vi "Setup voltage in.vi"(8 "error in (no error)":errorcluster, 10 "Run info in":T1, 11 "Sampling info in":T2={"Channels"=[], "Sampling freq"=0, "Output freq"=0, "Update freq"=0, "Steps per rev"=0, "Counts per rev"=0, "Amplifier"="", "Motor driver"="", "Step bit"=0, "Max speed"=0.0, "Max accel"=0.0, "Pos gain"=0.0, "Vel gain"=0.0, "counter"="Dev1/ctr0"} {"Channels"."Hi cutoff" items=["500"=500.0, "1k"=1000.0, "5k"=5000.0, "10k"=10000.0, "20k"=20000.0]; "Channels"."Lo cutoff" items=["0.1"=0.1, "1"=1.0, "10"=10.0, "100"=100.0, "300"=300.0]; "Channels"."Gain" items=["x100"=100, "x1000"=1000, "x10000"=10000]}) -> (0 "error out":errorcluster, 2 "Run info":T1, 3 "Sampling info out":T2={"Channels"=[], "Sampling freq"=0, "Output freq"=0, "Update freq"=0, "Steps per rev"=0, "Counts per rev"=0, "Amplifier"="", "Motor driver"="", "Step bit"=0, "Max speed"=0.0, "Max accel"=0.0, "Pos gain"=0.0, "Vel gain"=0.0, "counter"="Dev1/ctr0"} {"Channels"."Hi cutoff" items=["500"=500.0, "1k"=1000.0, "5k"=5000.0, "10k"=10000.0, "20k"=20000.0]; "Channels"."Lo cutoff" items=["0.1"=0.1, "1"=1.0, "10"=10.0, "100"=100.0, "300"=300.0]; "Channels"."Gain" items=["x100"=100, "x1000"=1000, "x10000"=10000]})   [LabVIEW 2012]
uses:
  Sampling info.ctl
  Channel.ctl
  Run info.ctl
  <vilib>/DAQmx/configure/timing.llb/DAQmx Timing (Sample Clock).vi
  <vilib>/DAQmx/create/channels.llb/DAQmx Create Channel (AI-Voltage-Basic).vi
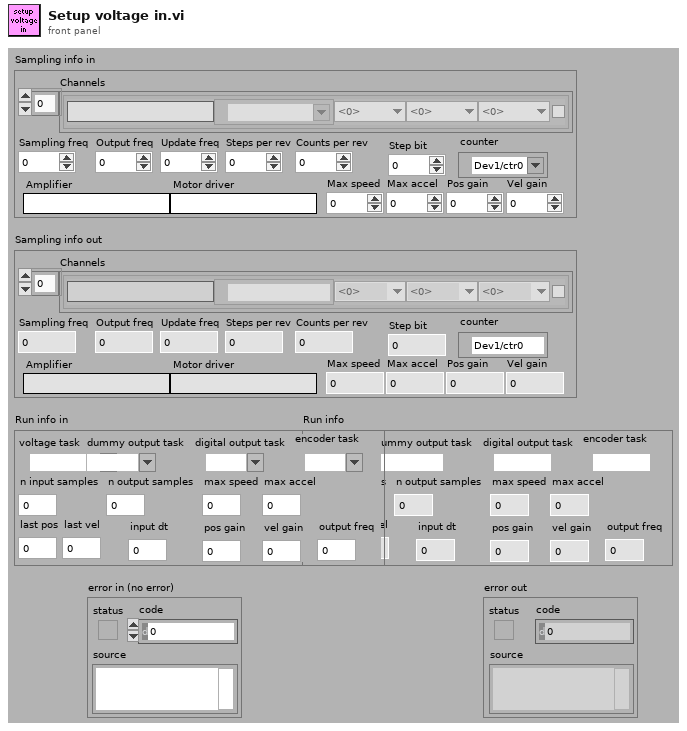
[diagram p1: front panel]
types:
  T1 = typedef "Run info.ctl" = cluster{"voltage task":refnum<k21>, "dummy output task":refnum<k21>, "digital output task":refnum<k21>, "encoder task":refnum<k21>, "n input samples":i32, "n output samples":i32, "max speed":dbl, "max accel":dbl, "last pos":dbl, "last vel":dbl, "pos gain":dbl, "vel gain":dbl, "input dt":dbl, "output freq":dbl}
  T2 = typedef "Sampling info.ctl" = cluster{"Channels":T3[], "Sampling freq":i32, "Output freq":i32, "Update freq":i32, "Steps per rev":i32, "Counts per rev":i32, "Amplifier":string, "Motor driver":string, "Step bit":u8, "Max speed":dbl, "Max accel":dbl, "Pos gain":dbl, "Vel gain":dbl, "counter":tag}
  T3 = typedef "Channel.ctl" = cluster{"Name":string, "Chan":tag, "Gain":u16, "Lo cutoff":dbl, "Hi cutoff":dbl, "Notch":bool}
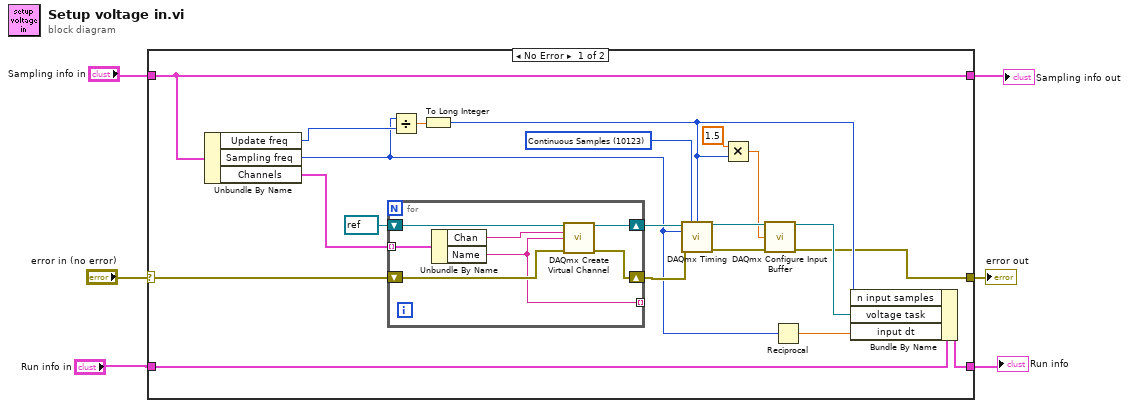
[diagram p0: block diagram]
diagram:
  n1 = case shown="No Error" "error in (no error)" {
    selector: "error in (no error)" -> [w24 w35]
    tunnel: [w23 w34] -> w2
    tunnel: [w9 w35] -> w5
    tunnel: [w25 w36] -> w1
    tunnel: "Sampling info in" -> [w25 w36]
    tunnel: "Run info in" -> [w22 w34]
    frame No Error {
      w18 = 10123 items=["Finite Samples"=10178, "Continuous Samples"=10123, "Hardware Timed Single Point"=12522] ("sample mode")
      n2 = Unbundle By Name(w25) -> ("Update freq"=w17:i32, "Sampling freq"=w8:i32, "Channels"=w21:T3[])
      n3 = for {
        tunnel: w21 -> [w33] mode=indexing
        shift-right: [w32] -> w20
        shift-left: refnum<k21> refnum ("task out") -> [w31]
        shift-right: [w28] -> w19
        shift-left: w24 -> [w29]
        tunnel: [w27] -> _ mode=indexing
        n4 = Unbundle By Name(w33) -> ("Chan"=w30:tag, "Name"=w27:string)
        n5 = call-poly <vilib>:"DAQmx Create Virtual Channel.vi"("task in"=w31, "physical channels"=w30, "name to assign"=w27, "error in"=w29) -> ("task out"=w32:refnum<k21>, "error out"=w28:errorcluster)  [unwired: 5 in, 5 out]
      }
      n6 = Divide(x=w8, y=w17) -> (x/y=w16:dbl)
      n7 = To Long Integer(number=w16) -> (32bit integer=w12:i32)
      n8 = call-poly <vilib>:"DAQmx Timing.vi"("task/channels in"=w20, "sample mode"=w18, "samples per channel"=w12, "rate"=w8, "error in"=w19) -> ("task out"=w15:refnum<k21>, "error out"=w14:errorcluster)  [unwired: 9 in]
      n9 = Multiply(x=1.5, y=w12) -> (x*y=w11:dbl)
      n10 = call <vilib>:"DAQmx Configure Input Buffer.vi"("task/channels in"=w15, "buffer size (in samples per channel)"=w11, "error in"=w14) -> ("task out"=w10:refnum<k21>, "error out"=w9:errorcluster)  [unwired: 11 in]
      n11 = Reciprocal(x=w8) -> (1/x=w7:dbl)
      n12 = Bundle By Name(cluster=w22, "n input samples"=w12, "voltage task"=w10, "input dt"=w7) -> (w23:T1)
    }
    frame Error {
    }
  }
  "error out" <- w5
  "Run info" <- w2
  "Sampling info out" <- w1
